vi "Destroy DVR.vi"(0 "HTTP GET Async ref in":refnum<data-value>, 11 "error in (no error)":errorcluster) -> (15 "error out":errorcluster)   [LabVIEW 2019, in "HTTP Client Extensions.lvlib" / "GET Async.lvclass"]
uses:
  GET Async.lvclass
  GET Async.lvclass/GET Async.ctl
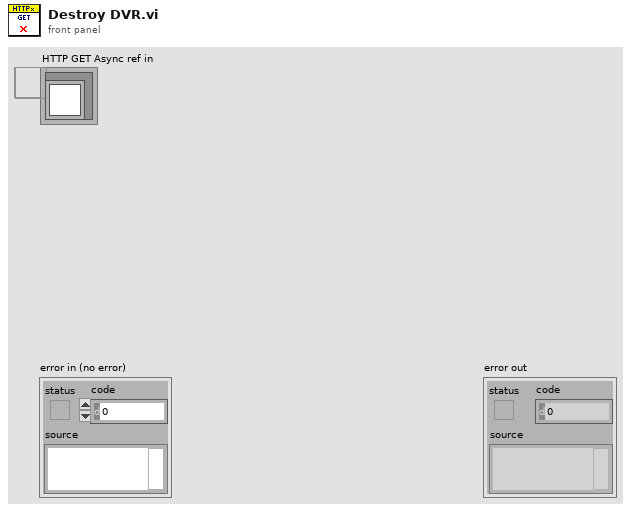
[diagram p1: front panel]
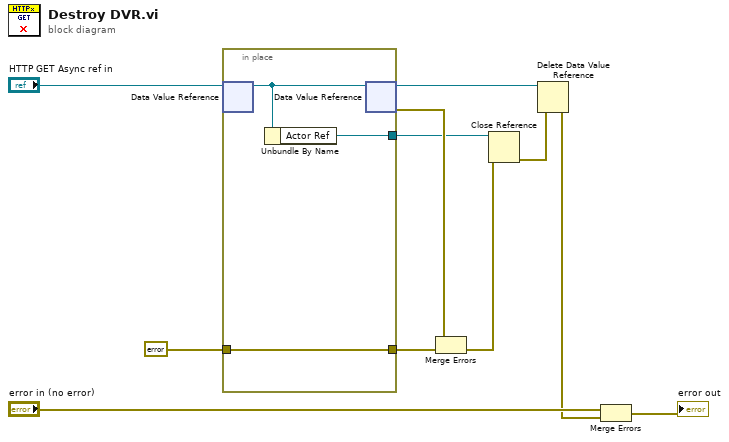
[diagram p0: block diagram]
diagram:
  n1 = in-place {
    in-place-border: errorcluster {"status"=FALSE, "code"=0, "source"=""} ("error in (no error)") -> [w13]
    in-place-border: [w13] -> w10
    in-place-border: [w12] -> w7
    n2 = in-place-dvr #1("HTTP GET Async ref in") -> (w14:refnum<class "GET Async.lvclass">)  [unwired: 1 out]
    n3 = Unbundle By Name(w14) -> ("Actor Ref"=w12:refnum<vi>)
    n4 = in-place-dvr #1(w14) -> (w6:refnum<data-value>, w9:errorcluster)
  }
  n5 = Merge Errors(w9, w10) -> (w4:errorcluster)
  n6 = Close Reference(reference=w7, error in (no error)=w4) -> (error out=w5:errorcluster)
  n7 = Delete Data Value Reference(data value reference=w6, error in=w5) -> (error out=w2:errorcluster)  [unwired: 1 out]
  n8 = Merge Errors("error in (no error)", w2) -> (→"error out":errorcluster)
